vi "Generator_Correlator.vi"() -> ()   [LabVIEW 2012]
uses:
  <vilib>/Utility/file.llb/Write To Spreadsheet File (DBL).vi
  RIGOL DG4000 Series/RIGOL DG4000 Series.lvlib
panel:
  out "Сдвиг на данном шаге":i64
  in  "Сколько точек\n сдвигать каждую итерацию 2":i32
  in  "Coincidence Sum Max n":i32
  out "Sum Coincidence Count N":i64
  out "Прошло итераций":i32
  in  "Количество различных сигналов диода":i32
  in  "Шаг ширины импульса":dbl format="%#.12p"
  in  "Путь":string="C:\\Измерения\\"
  out "Прошло итераций":i32
  out "Погрешность":cluster{"Y":dbl[], "Y":dbl[]}[](graph) caption="XY Graph 3"
  in  "Стартовый сдвиг":i16
  in  "Hight level (% of Counts)":dbl=0.15
  out "Измерения":cluster{"Y":dbl[], "Y":dbl[]}[](graph) caption="XY Graph 3"
  in  "Количество циклов измерений":i32
  out "Сигнал Диода":cluster{"Y":dbl[], "Y":dbl[]}[](graph) caption="XY Graph 3"
  in  "VISA resource name":refnum<visa-resource-name>="коррелятор"
  in  "Addr (0-15)":i8=1 min=0 max=15 step=1
  out "Measurement index":i64
  out "Total Afterpulsing Afterpulsing":i64
  out "Сдвиг на данном такте точек на данной итерации":i64
  in  "Сколько периодов копить":i16=1
  out "Measurement per takt":i64
  out "Coincidence Count SS1 control n":i64
  in  "Window Offset 1 (ns)":i32
  in  "Window Length 1 (ns)":i32
  in  "Start-Stop1 Multyplex":T1
  out "Single Count Channel1":i64
  out "Exposition time (ms)":i64
  in  "Ch1 Threshold V (mV)":i32=100 min=0 max=5000 step=10
  in  "Exposition Time (ms)":i64=1000
  in  "Коэффициент амплитуды":dbl format="%#_12f"
  in  "Ширина отрицательного импульса, тчк":dbl format="%#_12p"
  in  "Amplitude Unit (0: Vpp) 2":i32(ring) items=["Vpp", "Vrms", "dBm"]
  in  "Amplitude Диода (5 Vpp) 2":dbl=2.19
  in  "Amplitude Unit (0: Vpp)":i32(ring) items=["Vpp", "Vrms", "dBm"]
  in  "Amplitude Детектора (5 Vpp)":dbl=10.0
  in  "VISA":refnum<visa-resource-name>="USB0::0x1AB1::0x0641::DG4E184850441::INSTR"
  out "Разница между \nсигналом диода и детектора, с":dbl format="%.12p"
  in  "Сколько точек\n сдвигать каждую итерацию":i32
  in  "Время между импульсами, тчк 2":dbl format="%#_12p"
  in  "Ширина импульса, тчк":dbl=1e-06 format="%#_12p"
  in  "Количество точек":dbl=16000.0
  in  "Точек между импульсами, тчк":dbl format="%#_12p"
  in  "Точек в Ширина импульса, тчк":dbl=2.5e-07 format="%#_12p"
  out "Выход на канал 2":string
  out "Выход на канал 1":string
  in  "Частота (1000 Hz)":dbl=100000.0 format="%#_12p"
  # "ГЕНЕРАТОР"
  # "КОРРЕЛЯТОР"
  # "СИГНАЛЫ"
  # "ДЕТЕКТОР"
  # "ДИОД"
  # "Chanel 1"
  # "Chanel 2"
  # "Start from 0\n0 -> Channel1\n1 -> Channel2"
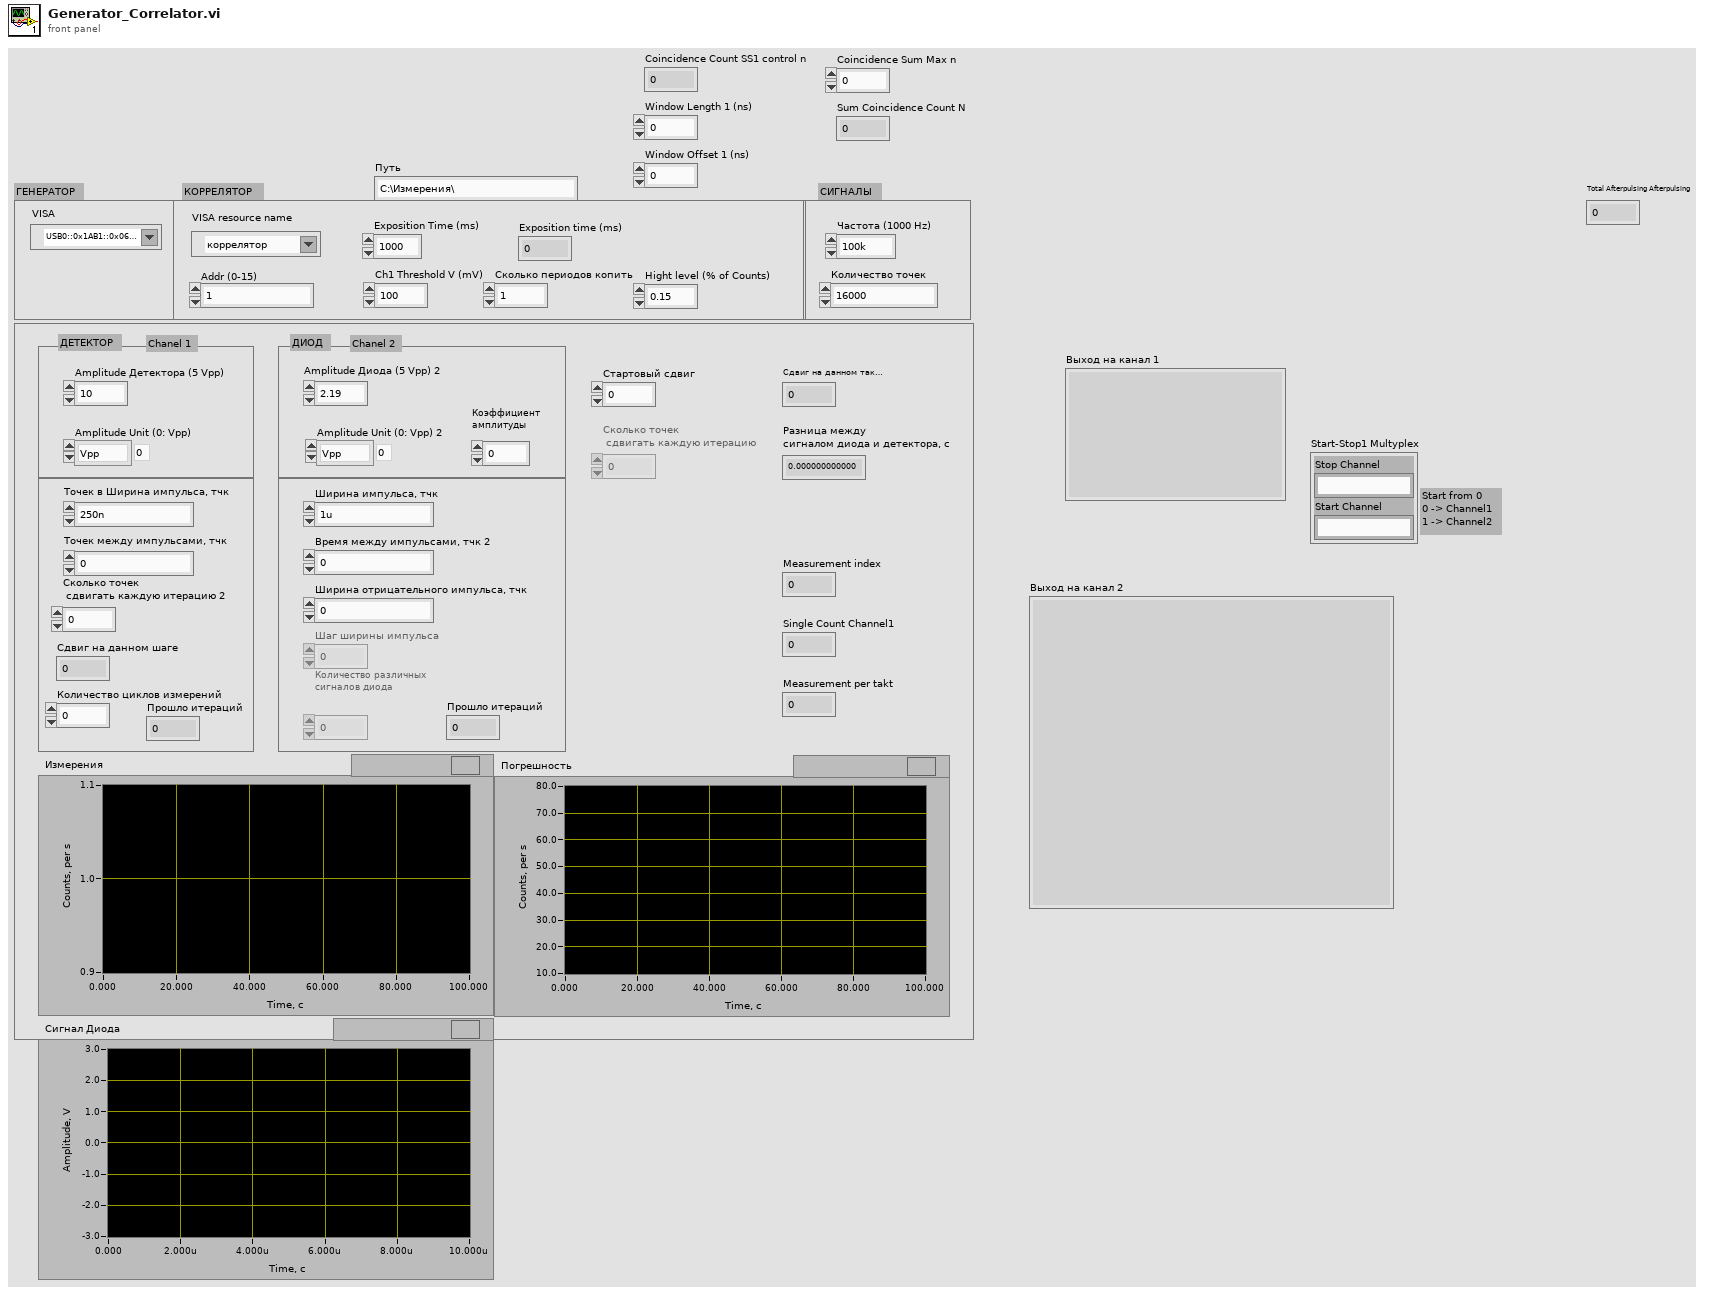
[diagram p1: front panel]
types:
  T1 = cluster{"Stop Channel":string, "Start Channel":string}
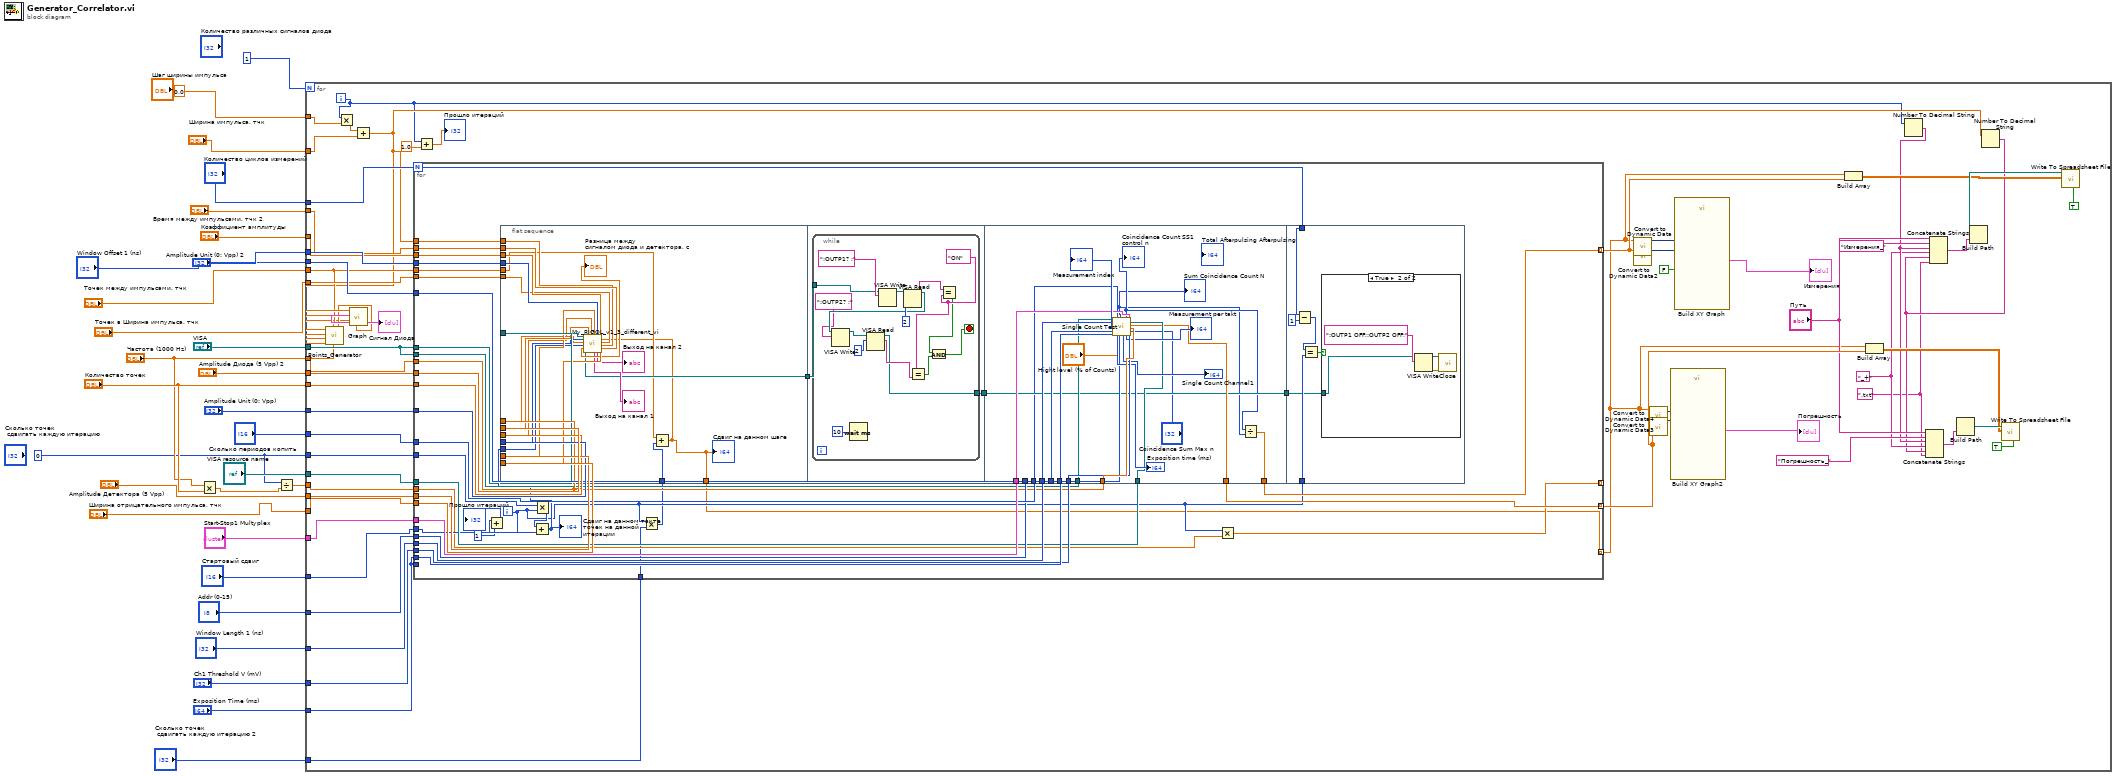
[diagram p0: block diagram]
diagram:
  w3 = 0 ("Сколько точек\n сдвигать каждую итерацию")
  n1 = Multiply(x="Частота (1000 Hz)", y="Количество точек") -> (x*y=w7:dbl)
  n2 = Divide(x=w3, y=w7) -> (x/y=w18:dbl)
  n3 = for {
    N: 1 ("Количество различных сигналов диода") -> [_]
    tunnel: "Amplitude Unit (0: Vpp) 2" -> [w88]
    tunnel: "Amplitude Unit (0: Vpp)" -> [w87]
    tunnel: "Время между импульсами, тчк 2" -> [w86]
    tunnel: "Start-Stop1 Multyplex" -> [w85]
    tunnel: "Ch1 Threshold V (mV)" -> [w84]
    tunnel: "Window Offset 1 (ns)" -> [w83]
    tunnel: "Window Length 1 (ns)" -> [w82]
    tunnel: "Addr (0-15)" -> [w81]
    tunnel: "VISA resource name" -> [w80]
    tunnel: "VISA" -> [w79]
    tunnel: "Amplitude Детектора (5 Vpp)" -> [w78]
    tunnel: w18 -> [w77]
    tunnel: "Сколько периодов копить" -> [w76]
    tunnel: "Exposition Time (ms)" -> [w75]
    tunnel: "Amplitude Диода (5 Vpp) 2" -> [w71]
    tunnel: "Точек в Ширина импульса, тчк" -> [w69]
    tunnel: "Точек между импульсами, тчк" -> [w67]
    tunnel: "Количество точек" -> [w66]
    tunnel: "Ширина отрицательного импульса, тчк" -> [w65]
    tunnel: "Коэффициент амплитуды" -> [w64]
    tunnel: "Количество циклов измерений" -> [w63]
    tunnel: "Частота (1000 Hz)" -> [w62]
    tunnel: w3 -> [w61]
    tunnel: "Стартовый сдвиг" -> [w59]
    tunnel: "Ширина импульса, тчк" -> [w42]
    tunnel: 0.0 ("Шаг ширины импульса") -> [w44]
    tunnel: "Сколько точек\n сдвигать каждую итерацию 2" -> [w31]
    i -> [w33]
    w37 = ".txt" ("string")
    w40 = "_+" ("string")
    n4 = Multiply(x=w33, y=w44) -> (x*y=w43:dbl)
    n5 = Add(x=w43, y=w42) -> (x+y=w39:dbl)
    n6 = call "Points_Generator.vi"("Частота (1000 Hz)"=w62, "Точек между импульсами, тчк in"=w67, "Коэффициент амплитуды"=w64, "Ширина отрицательного импульса, тчк in"=w65, "Количество точек in"=w66, "Ширина импульса, тчк in"=w39) -> ("Один импульс (диод)"=w68:dbl[])  [unwired: 5 out]
    n7 = call "Graph.vi"("Array"=w68, "Частота (1000 Hz)"=w62, "Количество точек"=w66, "Амплитуда"=w71) -> ("XY Graph 3"=→"Сигнал Диода":cluster{"Y":dbl[], "Y":dbl[]}[])  [unwired: 7 in]
    n8 = for {
      N: w63 -> [w107]
      tunnel: w64 -> [w128]
      tunnel: w65 -> [w127]
      tunnel: w71 -> [w126]
      tunnel: w78 -> [w125]
      tunnel: w88 -> [w124]
      tunnel: w87 -> [w123]
      tunnel: w62 -> [w108]
      tunnel: w69 -> [w122]
      tunnel: w67 -> [w121]
      tunnel: w79 -> [w99]
      tunnel: w86 -> [w120]
      tunnel: w39 -> [w119]
      tunnel: w66 -> [w118]
      tunnel: w85 -> [w116]
      tunnel: w84 -> [w111]
      tunnel: w75 -> [w113]
      tunnel: w83 -> [w112]
      tunnel: w82 -> [w114]
      tunnel: w76 -> [w115]
      tunnel: w61 -> [w117]
      tunnel: w81 -> [w110]
      tunnel: w80 -> [w109]
      tunnel: w79 -> [w106]
      tunnel: w77 -> [w101]
      tunnel: w75 -> [_]
      tunnel: [w100] -> _ mode=indexing
      tunnel: [w93] -> w52 mode=indexing
      tunnel: w59 -> [w103]
      tunnel: [w102] -> w48 mode=indexing
      tunnel: w31 -> [w92]
      tunnel: [w89] -> w30 mode=indexing
      i -> [w91]
      n9 = Add(x=w91, y=1) -> (x+y=→"Прошло итераций":i32)
      n10 = flat-sequence {
        tunnel: w128 -> [w148]
        tunnel: w127 -> [w147]
        tunnel: w126 -> [w146]
        tunnel: w125 -> [w145]
        tunnel: w124 -> [w143]
        tunnel: w123 -> [w142]
        tunnel: w108 -> [w141]
        tunnel: w122 -> [w140]
        tunnel: w121 -> [w130]
        tunnel: w99 -> [w139]
        tunnel: w120 -> [w138]
        tunnel: w119 -> [w137]
        tunnel: w118 -> [w136]
        tunnel: w105 -> [w133]
        tunnel: [w132] -> w98
        tunnel: w90 -> [w131]
        tunnel: [w129] -> w89
        tunnel: w98 -> [w150]
        tunnel: [w149] -> w96
        tunnel: w116 -> [w176]
        tunnel: w115 -> [w171]
        tunnel: w114 -> [w179]
        tunnel: w113 -> [w182]
        tunnel: w112 -> [w181]
        tunnel: w111 -> [w186]
        tunnel: w110 -> [w177]
        tunnel: w109 -> [w175]
        tunnel: w106 -> [w178]
        tunnel: w108 -> [w187]
        tunnel: [w173] -> w102
        tunnel: [w172] -> w97
        tunnel: w96 -> [w172]
        tunnel: [w167] -> w93
        tunnel: w91 -> [w192]
        tunnel: w107 -> [w191]
        tunnel: w97 -> [w188]
        frame #0 {
          n11 = Add(x=w130, y=w131) -> (x+y=w129:dbl)
          "Сдвиг на данном шаге" <- w129
          n12 = call "My_RIGOL_v1_3_different_vi.vi"("VISA"=w139, "Amplitude Unit (0: Vpp)"=w142, "Частота (1000 Hz)"=w141, "Сколько точек\n сдвигать"=w133, "Amplitude Диода (5 Vpp) 2"=w146, "Количество точек"=w136, "Amplitude Детектора (5 Vpp)"=w145, "Amplitude Unit (0: Vpp) 2"=w143, "Коэффициент амплитуды"=w148, "Точек между импульсами, тчк"=w129, "Ширина импульса, тчк"=w140, "Ширина импульса, с 2"=w137, "Время между импульсами, с 2"=w138, "Ширина отрицательного импульса, с"=w147) -> ("Разница между \nсигналом диода и детектора, с"=→"Разница между \nсигналом диода и детектора, с":dbl, "VISA resource name out"=w132:refnum<visa-resource-name>, "Выход на канал 1"=→"Выход на канал 1":string, "Выход на канал 2"=→"Выход на канал 2":string)  [unwired: 2 out]
        }
        frame #1 {
          n13 = while {
            tunnel: w150 -> [w161]
            tunnel: [w151] -> w149
            stop <- w152 stop-if-true
            w155 = "ON"
            n14 = Wait (ms)(milliseconds to wait=u32 10) -> ()  [unwired: 1 out]
            n15 = VISA Write(VISA resource name=w161, write buffer=":OUTP1? ;") -> (VISA resource name out=w165:refnum<visa-resource-name>)  [unwired: 1 in, 2 out]
            n16 = VISA Read(VISA resource name=w165, byte count=u32 2) -> (VISA resource name out=w160:refnum<visa-resource-name>, read buffer=w162:string)  [unwired: 1 in, 2 out]
            n17 = VISA Write(VISA resource name=w160, write buffer=":OUTP2? ;") -> (VISA resource name out=w159:refnum<visa-resource-name>)  [unwired: 1 in, 2 out]
            n18 = VISA Read(VISA resource name=w159, byte count=u32 2) -> (VISA resource name out=w151:refnum<visa-resource-name>, read buffer=w156:string)  [unwired: 1 in, 2 out]
            n19 = Equal?(x=w155, y=w156) -> (x = y?=w153:bool)
            n20 = Equal?(x=w162, y=w155) -> (x = y?=w154:bool)
            n21 = And(x=w154, y=w153) -> (x .and. y?=w152:bool)
          }
        }
        frame #2 {
          n22 = call "Single Count Test.vi"("VISA resource name generator 2"=w178, "Window Length 1 (ns)"=w179, "Window Offset 1 (ns)"=w181, "Exposition Time (ms)"=w182, "Сколько периодов копить"=w171, "Hight level (% of Counts)"="Hight level (% of Counts)", "Addr (0-15)"=w177, "Start-Stop1 Multyplex"=w176, "VISA resource name"=w175, "Частота (1000 Hz)"=w187, "Coincidence Sum Max n"="Coincidence Sum Max n", "Channel1 Threshold Voltage (mV)"=w186) -> ("Measurement index"=→"Measurement index":i64, "Exposition time (ms)  то, что нужно"=→"Exposition time (ms)":i64, "Sum Coincidence Count N"=w168:i64, "Single Count Channel1"=→"Single Count Channel1":i64, "Coincidence Count SS1 n control"=w169:i64, "Total"=→"Measurement per takt":i64, "delta error"=w173:dbl)  [unwired: 1 out]
          "Coincidence Count SS1 control n" <- w169
          "Sum Coincidence Count N" <- w168
          n23 = Divide(x=w169, y=w168) -> (x/y=w167:dbl)
        }
        frame #3 {
          n24 = Subtract(x=w191, y=1) -> (x-y=w189:i32)
          n25 = Equal?(x=w189, y=w192) -> (x = y?=w193:bool)
          n26 = case shown="True" w193 {
            tunnel: w188 -> [_ w194]
            frame False {
            }
            frame True {
              n27 = VISA Write(VISA resource name=w194, write buffer=":OUTP1 OFF;:OUTP2 OFF;") -> (VISA resource name out=w196:refnum<visa-resource-name>, error out=w195:errorcluster)  [unwired: 1 in, 1 out]
              n28 = call "Close.vi"("error in (no error)"=w195, "VISA resource name"=w196) -> ()  [unwired: 10 out]
            }
          }
        }
      }
      n29 = Multiply(x=w117, y=w91) -> (x*y=w104:i32)
      n30 = Add(x=w104, y=w103) -> (x+y=w105:i32)
      "Сдвиг на данном такте точек на данной итерации" <- w105
      n31 = Multiply(x=w91, y=w92) -> (x*y=w90:i32)
      n32 = Multiply(x=w91, y=w101) -> (x*y=w100:dbl)
    }
    n33 = Add(x=w33, y=1.0) -> (x+y=→"Прошло итераций":dbl)
    n34 = call "Convert to Dynamic Data"("Array"=w30) -> ("Dynamic Data Type"=w74:dynamicdata)  [unwired: 3 in]
    n35 = call "Convert to Dynamic Data2"("Array"=w52) -> ("Dynamic Data Type"=w73:dynamicdata)  [unwired: 3 in]
    n36 = call "Convert to Dynamic Data4"("Array"=w30) -> ("Dynamic Data Type"=w57:dynamicdata)  [unwired: 3 in]
    n37 = call "Convert to Dynamic Data3"("Array"=w48) -> ("Dynamic Data Type"=w58:dynamicdata)  [unwired: 3 in]
    n38 = call "Build XY Graph2"("Y Input"=w58, "X Input"=w57) -> ("XY Graph"=→"Погрешность":cluster{"Y":dbl[], "Y":dbl[]}[])  [unwired: 3 in, 6 out]
    n39 = call "Build XY Graph"("Reset"=FALSE, "Y Input"=w73, "X Input"=w74) -> ("XY Graph"=→"Измерения":cluster{"Y":dbl[], "Y":dbl[]}[])  [unwired: 2 in, 6 out]
    n40 = Build Array(w30, w52) -> (w53:dbl[][])
    n41 = Build Array(w30, w48) -> (w49:dbl[][])
    n42 = Number To Decimal String(number=w33) -> (decimal integer string=w41:string)  [unwired: 1 in]
    n43 = Number To Decimal String(number=w39) -> (decimal integer string=w38:string)  [unwired: 1 in]
    n44 = Concatenate Strings("Путь", "Погрешность_" ("string"), w41, w40, w38, w37) -> (w35:string)
    n45 = Concatenate Strings("Путь", "Измерения_" ("string"), w41, w40, w38, w37) -> (w36:string)
    n46 = Build Path(name or relative path=w35) -> (appended path=w50:path)  [unwired: 1 in]
    n47 = Build Path(name or relative path=w36) -> (appended path=w54:path)  [unwired: 1 in]
    n48 = call-poly <vilib>:"Write To Spreadsheet File.vi"("transpose? (no:F)"=TRUE, "2D data"=w49, "file path (dialog if empty)"=w50) -> ()  [unwired: 5 in, 1 out]
    n49 = call-poly <vilib>:"Write To Spreadsheet File.vi"("transpose? (no:F)"=TRUE, "2D data"=w53, "file path (dialog if empty)"=w54) -> ()  [unwired: 5 in, 1 out]
  }
